vi "Terminate.vi"(8 "error in (no error)":errorcluster, 10 "Message in":refnum<class "TerminateMessage.lvclass">, 11 "StageSPIM in":refnum<class "StageSPIM.lvclass">) -> (0 "error out":errorcluster, 3 "StageSPIM out":refnum<class "StageSPIM.lvclass">)   [LabVIEW 2012, in "StageSPIM.lvclass"]
doc: "This member function is called when the statemachine in the run.vi receives an 'terminate' command. It closes the RabbitMQ connection. \n\nOverride this member function in your derived class to release all previously acquired resources (but don't forget to call the parent method). If your component has subcomponents, they count as resources, and you have to release them by calling their own terminate functions."
uses:
  StageSPIM.lvclass
  <vilib>/Distrio/Murmex/TerminateMessage/TerminateMessage.lvclass
  StageSPIM.lvclass/StageSPIM.ctl
  <vilib>/Distrio/Murmex/Murmex/Murmex.lvclass
panel:
  out "Array":bool[](array[boolean])
  # "This method is called when the TERMINATE\ntrigger is sent. \n\nOverride this method when your component needs to\nrespond to this trigger. \n\nCall parent for proper implementation"
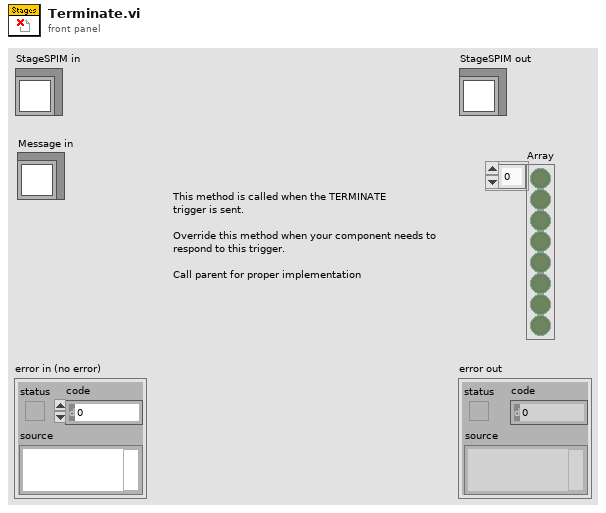
[diagram p1: front panel]
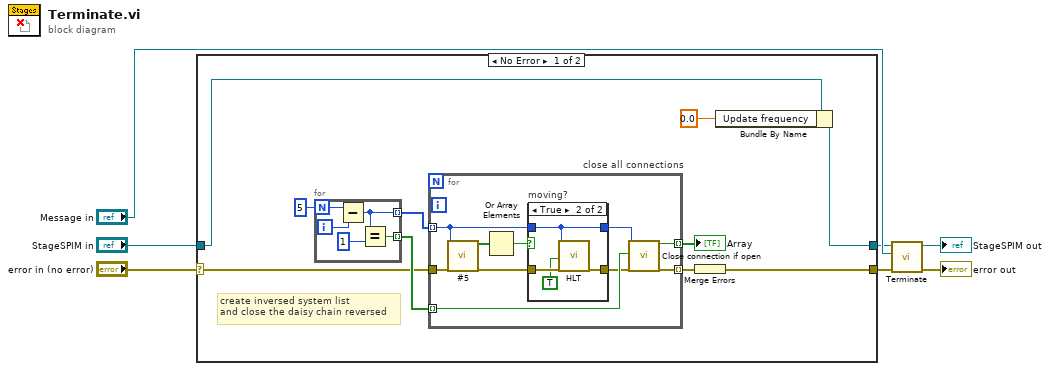
[diagram p0: block diagram]
diagram:
  n1 = case shown="No Error" "error in (no error)" {
    selector: "error in (no error)" -> [w12 w39]
    tunnel: [w11 w39] -> w5
    tunnel: "StageSPIM in" -> [w10 w40]
    tunnel: [w9 w40] -> w1
    frame No Error {
      # "create inversed system list\nand close the daisy chain reversed"
      n2 = for {
        N: 5 -> [w22]
        tunnel: [w20] -> w15 mode=indexing
        tunnel: [w18] -> w14 mode=indexing
        i -> [w21]
        n3 = Subtract(x=w22, y=w21) -> (x-y=w20:i32)
        n4 = Equal?(x=w20, y=1) -> (x = y?=w18:bool)
      }
      n5 = for "close all connections" {
        tunnel: w15 -> [w28] mode=indexing
        tunnel: w14 -> [w32] mode=indexing
        tunnel: [w31] -> w17 mode=indexing
        tunnel: w12 -> [w27]
        tunnel: [w30] -> w16 mode=indexing
        n6 = call "#5.vi"("System no."=w28, "error in"=w27) -> ("Axis moving?"=w25:bool[], "error out"=w26:errorcluster)  [unwired: 16 in]
        n7 = Or Array Elements(Boolean array=w25) -> (logical OR=w24:bool)
        n8 = case "moving?" shown="True" w24 {
          tunnel: [w33 w38] -> w29
          tunnel: w28 -> [w34 w35]
          tunnel: w26 -> [w33 w37]
          tunnel: [w34 w35] -> w23
          frame False {
          }
          frame True {
            n9 = call "HLT.vi"("System no."=w35, "All axes?"=TRUE ("all axes"), "error in"=w37) -> ("error out"=w38:errorcluster)  [unwired: 16 in]
          }
        }
        n10 = call "Close connection if open.vi"("System no."=w23, "Close DaisyChain"=w32, "error in"=w29) -> ("Was connected?"=w31:bool, "error out"=w30:errorcluster)  [unwired: 15 in]
      }
      "Array" <- w17
      n11 = Merge Errors(w16) -> (w11:errorcluster)
      n12 = Bundle By Name(cluster=w10, "Update frequency"=dbl[unit] 0.0 ("configuration.Update frequency")) -> (w9:refnum<class "StageSPIM.lvclass">)
    }
    frame Error {
    }
  }
  n13 = call-parent "Terminate.vi"("error in (no error)"=w5, "Message in"="Message in", "Murmex in"=w1) -> ("error out"=→"error out":errorcluster, "Murmex out"=→"StageSPIM out":refnum<class "StageSPIM.lvclass">)  [unwired: 7 in]
